vi "Handle Menu Selection.vi"(4 "SubObj":refnum<vi>, 5 "VolatusAPI":refnum<class "VolatusAPI.lvclass">, 6 "Coords":T1, 7 "CtlRef":refnum<vi>, 8 "error in (no error)":errorcluster, 9 "ItemPath":string, 10 "ItemTag":string, 11 "OnShortcutMenuHandler in":refnum<class "OnShortcutMenuHandler.lvclass">) -> (0 "error out":errorcluster, 3 "OnShortcutMenuHandler out":refnum<class "OnShortcutMenuHandler.lvclass">)   [LabVIEW 2020, in "VolatusGUI.lvlib" / "OnShortcutMenuHandler.lvclass"]
uses:
  OnShortcutMenuHandler.lvclass
  <vilib>/Utility/miscctls.llb/LVPoint32TypeDef.ctl
  Volatus/VolatusAPI/VolatusAPI.lvclass
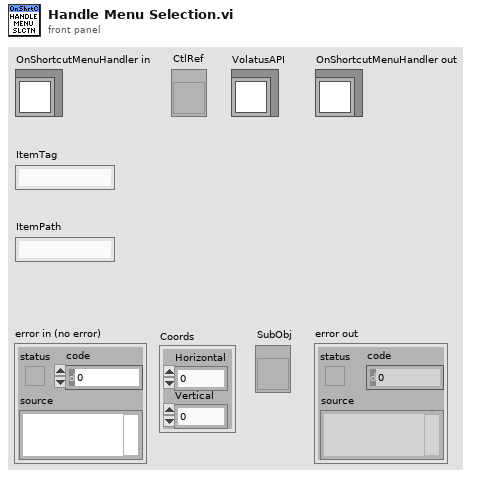
[diagram p1: front panel]
types:
  T1 = typedef "LVPoint32TypeDef.ctl" = cluster{"Horizontal":i32, "Vertical":i32}
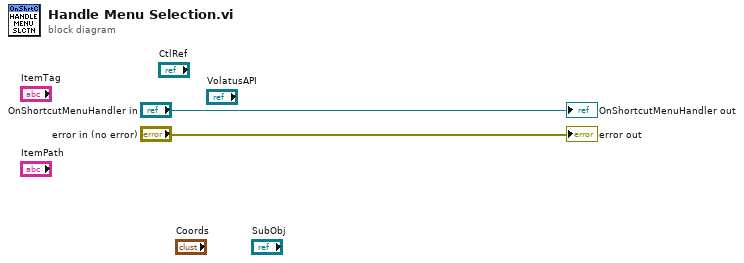
[diagram p0: block diagram]
diagram:
  "error out" <- "error in (no error)"
  "OnShortcutMenuHandler out" <- "OnShortcutMenuHandler in"
